vi "get_commandQueue.vi"(8 "error in (no error)":errorcluster, 11 "HGF_SVMonitor.lvclass in":refnum<class "HGF_SVMonitor.lvclass">) -> (0 "error out":errorcluster, 2 "command queue":refnum<queue>, 3 "HGF_SVMonitor.lvclass out":refnum<class "HGF_SVMonitor.lvclass">)   [LabVIEW 2009]
uses:
  HGF_SVMonitor.lvclass
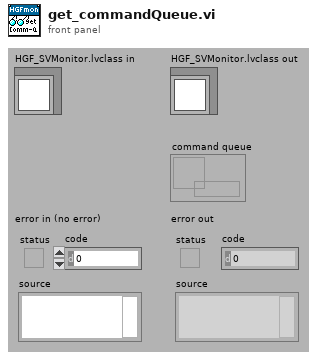
[diagram p1: front panel]
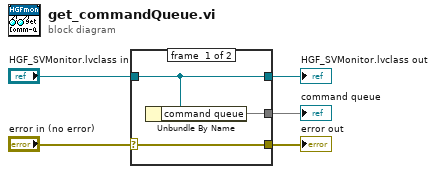
[diagram p0: block diagram]
diagram:
  n1 = case shown="No Error" "error in (no error)" {
    selector: "error in (no error)" -> [w8 w9]
    tunnel: [w8 w9] -> w4
    tunnel: [w7 w10] -> w2
    tunnel: "HGF_SVMonitor.lvclass in" -> [w7 w10]
    tunnel: [w6 _] -> w1
    frame #0 {
      n2 = Unbundle By Name(w7) -> ("command queue"=w6)
    }
    frame #1 {
    }
  }
  "error out" <- w4
  "HGF_SVMonitor.lvclass out" <- w2
  "command queue" <- w1
